vi "Run JSL Script.vi"   [LabVIEW 2019, in "JMP Automation.lvlib"]
doc: "Run a JSL script from a string or from a file depending of the polymorphic form selected"
uses:
  JMP Automation.lvlib
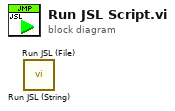
[diagram p0: block diagram]
diagram:
  n1 = call "Run JSL (String).vi"() -> ()  [unwired: 10 in, 2 out]
  n2 = call "Run JSL (File).vi"() -> ()  [unwired: 10 in, 2 out]
